vi "Read Action.vi"(8 "error in (no error)":errorcluster, 11 "EventsAbstract in":refnum<class "EventsAbstract.lvclass">) -> (0 "error out":errorcluster, 2 "Action":T1, 3 "EventsAbstract out":refnum<class "EventsAbstract.lvclass">)   [LabVIEW 2019, in "EventsAbstract.lvclass"]
uses:
  EventsAbstract.lvclass
  Modules/ModuleAbstract/TypeDef/Module Actions.ctl
  EventsAbstract.lvclass/EventsAbstract.ctl
  Modules/ModuleAbstract/ModuleAbstract.lvclass
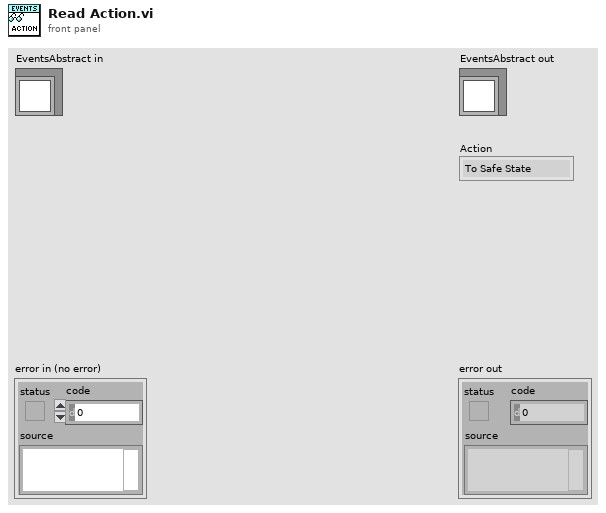
[diagram p1: front panel]
types:
  T1 = typedef "ModuleAbstract.lvlib/ModuleAbstract.lvclass/Module Actions.ctl" = enum16{"To Safe State", "Reset Safe State", "Close Module"}
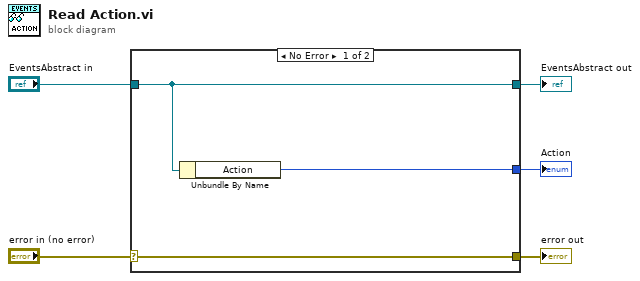
[diagram p0: block diagram]
diagram:
  n1 = case shown="No Error" "error in (no error)" {
    selector: "error in (no error)" -> [w8 w9]
    tunnel: [w8 w9] -> w4
    tunnel: [w7 w10] -> w2
    tunnel: "EventsAbstract in" -> [w7 w10]
    tunnel: [w6 _] -> w1
    frame No Error {
      n2 = Unbundle By Name(w7) -> ("Action"=w6:T1)
    }
    frame Error {
    }
  }
  "error out" <- w4
  "EventsAbstract out" <- w2
  "Action" <- w1
